vi "Sensor Interface View.vi"(8 "error in (no error)":errorcluster, 11 "View Model":T1) -> (0 "error out":errorcluster)   [LabVIEW 2017]
doc: "The interface where a user changes the floor location of the Elevator.\n[Covers: UI4]"
uses:
  View Model/Controls/View Model.ctl
  View Model/Controls/Shared Model.ctl
  Error Handler/Controls/Error Model.ctl
  Error Handler/Controls/Error Data.ctl
  Error Handler/Controls/Error Level.ctl
  Configuration/Controls/Config Model.ctl
  Configuration/Controls/Config Data Record.ctl
  Configuration/Controls/Config Command.ctl
  Controller/Controls/Control Model.ctl
  Controller/Controls/Elevator Location.ctl
  Controller/Controls/Elevator Status.ctl
  Controller/Controls/Control Event.ctl
  Controller/Controls/Control CMD.ctl
panel:
  out "Elevator Position":u16(slide)=1 min=1 max=4 step=1 scale=1.0..4.0
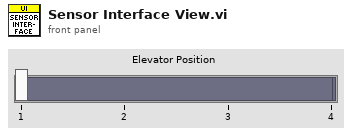
[diagram p1: front panel]
types:
  T1 = typedef "View Model.ctl" = cluster{"Shared Model":T2, "Error Model":T3, "Config Model":T4, "Control Model":T5}
  T2 = typedef "Shared Model.ctl" = cluster{"Stop":refnum<user-event>, "Stop DVR":refnum<data-value>}
  T3 = typedef "Error Model.ctl" = cluster{"Error":refnum<user-event>}
  T4 = typedef "Config Model.ctl" = cluster{"Data DVR":refnum<data-value>, "Config CMD":refnum<user-event>}
  T5 = typedef "Control Model.ctl" = cluster{"Location Change":refnum<user-event>, "Location DVR":refnum<data-value>, "Elapsed Time DVR":refnum<data-value>, "Direction Change":refnum<user-event>, "Door Posit Change":refnum<user-event>, "Emergency Change":refnum<user-event>, "Status Change":refnum<user-event>, "Status DVR":refnum<data-value>, "Command":refnum<user-event>}
  T6 = typedef "Elevator Location.ctl" = enum16{"1st Floor", "2nd Floor", "3rd Floor", "4th Floor"}
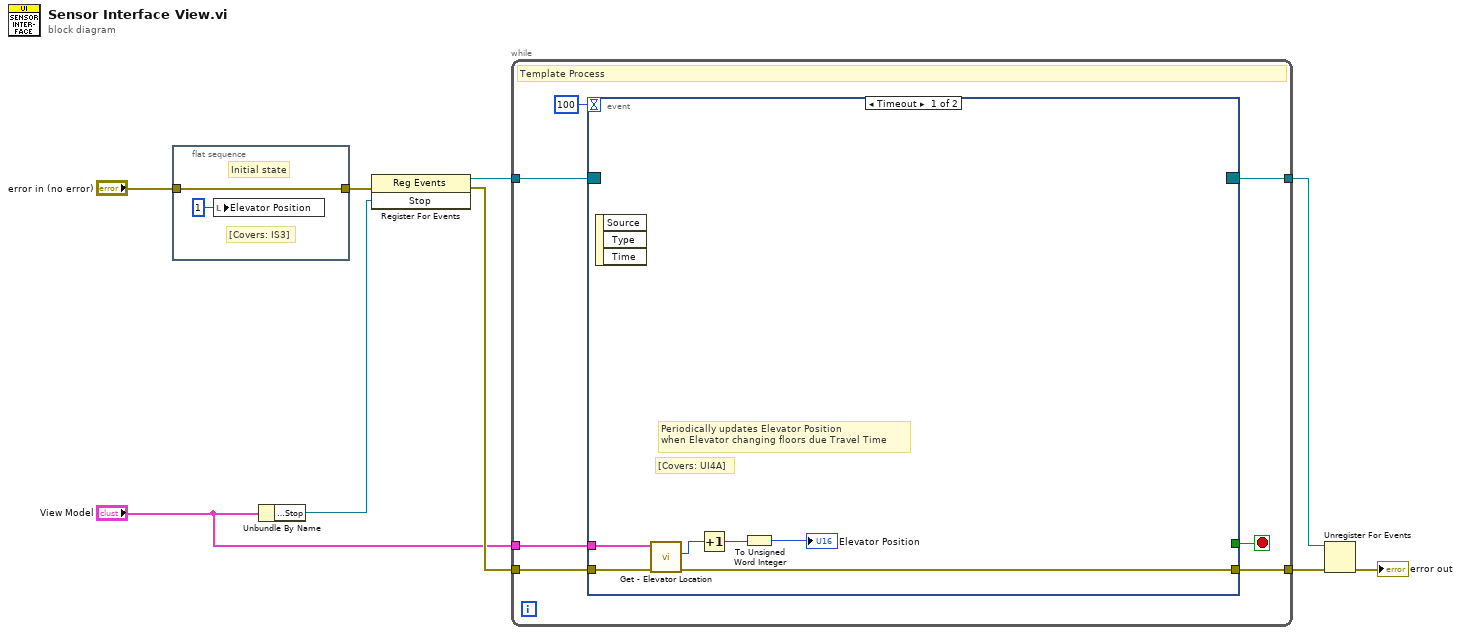
[diagram p0: block diagram]
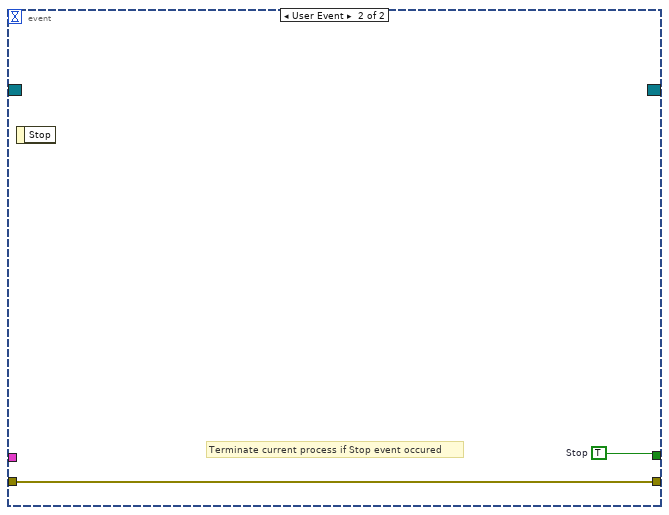
[diagram p2: hidden frame]
diagram:
  n1 = flat-sequence {
    tunnel: [w10] -> w1
    tunnel: "error in (no error)" -> [w10]
    frame #0 {
      # "[Covers: IS3]"
      # "Initial state"
      n2 = local write "Elevator Position"(u16 1 ("Elevator Position")) -> ()
    }
  }
  n3 = Unbundle By Name("View Model") -> ("Shared Model.Stop"=w9:refnum<user-event>)
  n4 = register-events(error in=w1, w9) -> (reference out=w8:refnum<event-registration>, error out=w7:errorcluster)  [unwired: 1 in]
  n5 = while {
    tunnel: w8 -> [w18]
    tunnel: w7 -> [w17]
    tunnel: [w16] -> w5
    tunnel: [w14] -> w6
    tunnel: "View Model" -> [w12]
    stop <- w15 stop-if-true
    # "Template Process"
    n6 = event shown="[0] Timeout" {
      selector: w18 -> [_ _]
      dyn-events: [_ _] -> w14
      timeout: 100 -> [_ _]
      tunnel: w17 -> [w24 w26]
      tunnel: [w23 w26] -> w16
      tunnel: [_ w25] -> w15
      tunnel: w12 -> [w22 _]
      event Timeout {
        # "[Covers: UI4A]"
        # "Periodically updates Elevator Position\nwhen Elevator changing floors due Travel Time"
        n7 = event-data() -> ()  [unwired: 1 in, 3 out]
        n8 = call "Get - Elevator Location.vi"("error in (no error)"=w24, "View Model"=w22) -> ("error out"=w23:errorcluster, "Elevator Location"=w19:T6)  [unwired: 7 in, 1 out]
        n9 = Increment(x=w19) -> (x+1=w21:T6)
        n10 = To Unsigned Word Integer(number=w21) -> (unsigned 16bit integer=→"Elevator Position":u16)
      }
      event User Event {
        w25 = TRUE  # Stop
        # "Terminate current process if Stop event occured"
        n11 = event-data() -> ()  [unwired: 1 in, 1 out]
      }
    }
  }
  n12 = Unregister For Events(event registration refnum=w6, error in=w5) -> (error out=→"error out":errorcluster)
